vi "Main(Analysis_Debug2_Mode).vi"() -> ()   [LabVIEW 2015]
panel:
  in  "Use Filter data":bool
  in  "Use Time Range":bool
  in  "Data Range Subset":bool
  in  "Time Range(SEC)":dbl
  in  "Analysis List":i32(listbox)
  in  "Data Range Addition":bool
  in  "Over-write":bool
  in  "Number of Data Down-Sampling":dbl
  in  "Save As":bool
  in  "Refresh":bool
  in  "Delete":bool
  in  "Plot Style":string(combo)
  in  "File Name":string(combo)
  in  "Analysis mode":enum16{""}(ring)
  in  "확인 버튼":bool
  in  "File Path":path
  out "XY 그래프":cluster{"Time(s)":dbl[], "calculation":u32[]}[](graph)
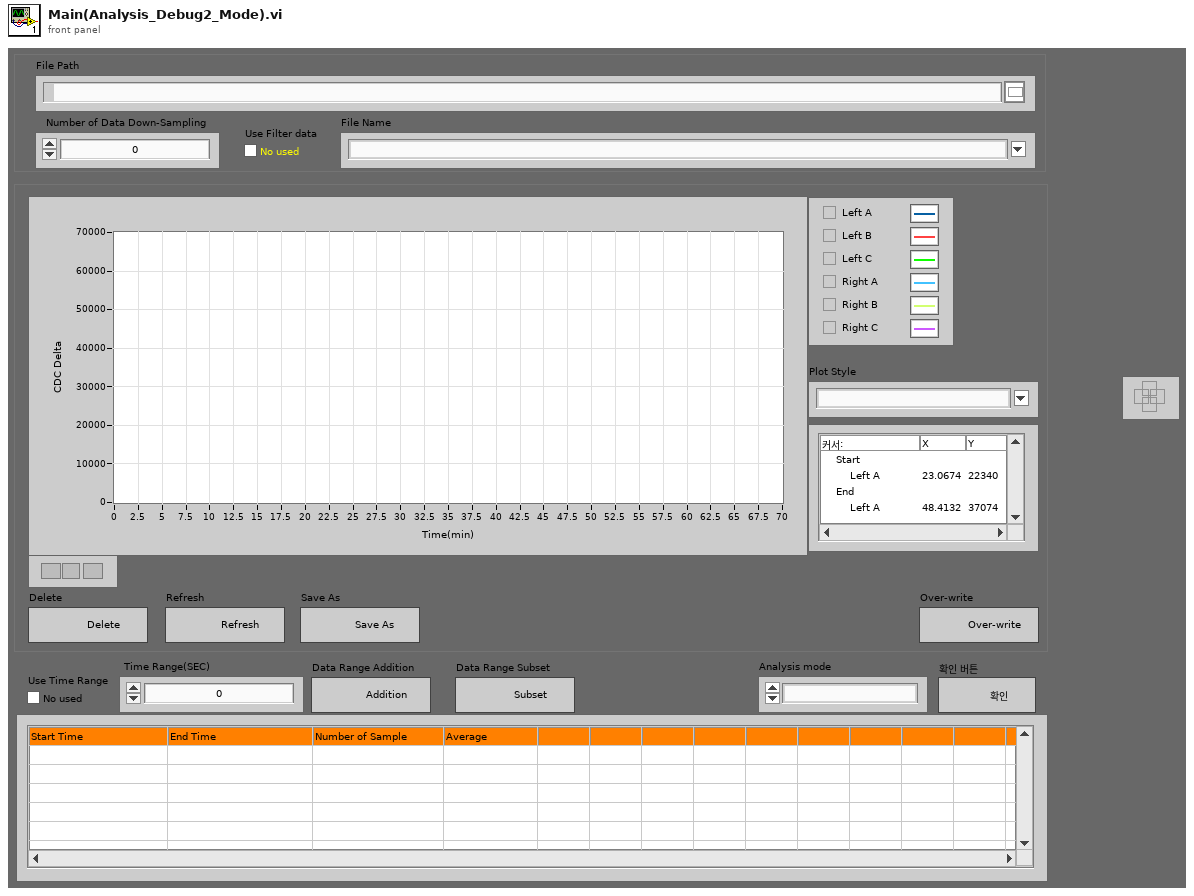
[diagram p1: front panel]
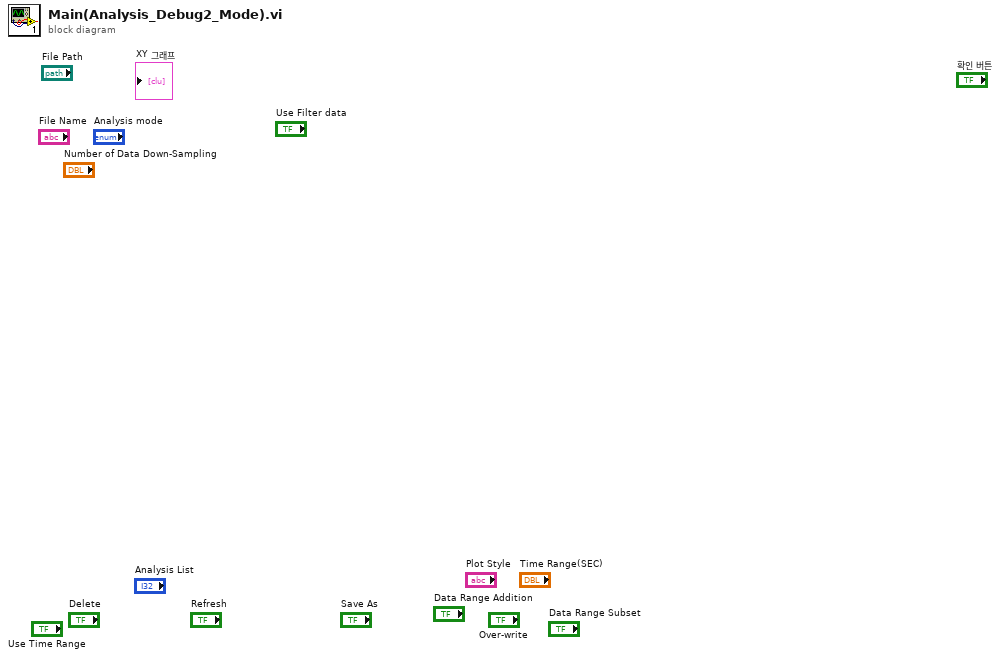
[diagram p0: block diagram]
diagram:
